vi "Table_Add_ShowNew.vi"(6 "数据输入":string[](array[string]), 7 "Tbl引用句柄":refnum<vi>) -> ()   [LabVIEW 2019]
panel:
  # "将数据加入表格，并显示到最新的显示处"
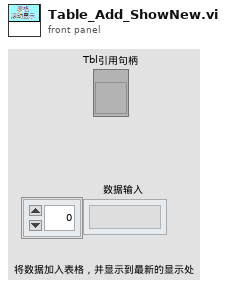
[diagram p1: front panel]
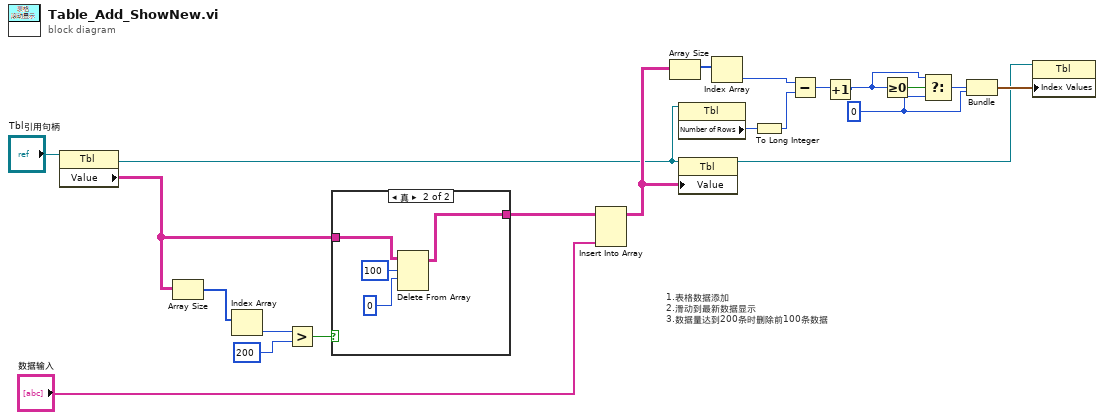
[diagram p0: block diagram]
diagram:
  w13 = 0 ("f")
  # "1.表格数据添加\n2.滑动到最新数据显示\n3.数据量达到200条时删除前100条数据"
  n1 = property class="Tbl"(reference="Tbl引用句柄") -> (reference out=w8:refnum<vi>, "Value"=w2:string[][])  [unwired: 1 in, 1 out]
  n2 = Array Size(array=w2) -> (size(s)=w6:i32[])
  n3 = Index Array(array=w6) -> (element=w5:i32)  [unwired: 1 in]
  n4 = Greater?(x=w5, y=200) -> (0:w3:bool)
  n5 = case shown="真" w3 {
    tunnel: w2 -> [w22 w26]
    tunnel: [w22 w23] -> w1
    frame False {
    }
    frame True {
      n6 = Delete From Array(array=w26, length=100 ("长度"), index (row)=0 ("索引 (行)")) -> (array with subset deleted=w23:string[][])  [unwired: 1 in, 1 out]
    }
  }
  n7 = Insert Into Array(array=w1, new element="数据输入") -> (w10:string[][])  [unwired: 2 in]
  n8 = Array Size(array=w10) -> (size(s)=w18:i32[])
  n9 = property on="属性节点" class="Tbl"(reference=w8) -> ("Number of Rows"=w12:u32)  [unwired: 1 in, 2 out]
  n10 = property class="Tbl"(reference=w8, "Value"=w10) -> (reference out=w7:refnum<vi>)  [unwired: 1 in, 1 out]
  n11 = Index Array(array=w18) -> (element=w17:i32)  [unwired: 1 in]
  n12 = To Long Integer(number=w12) -> (32bit integer=w11:i32)
  n13 = Subtract(x=w17, y=w11) -> (x-y=w15:i32)
  n14 = Increment(x=w15) -> (x+1=w14:i32)
  n15 = Greater Or Equal To 0?(x=w14) -> (x >= 0?=w20:bool)
  n16 = Select(t=w14, s=w20, f=w13) -> (s? t:f=w19:i32)
  n17 = Bundle("f"=w19, "f"=w13) -> (w16:cluster{"f":i32, "f":i32})  [unwired: 1 in]
  n18 = property on="属性节点" class="Tbl"(reference=w7, "Index Values"=w16) -> ()  [unwired: 1 in, 2 out]
